vi "Length_14.vi"() -> ()   [LabVIEW 2020]
uses:
  Support/Controls/Cmd_Mouse Popup.ctl
  Support/Controls/Clst_Initialize Input.ctl
  Support/Controls/Cmd_Var Data IO.ctl
  Variables/Global_Cal Info.vi
  Support/Public/Polymorph/Rmv Empt Arr_1D Str.vi
  Support/Public/Polymorph/Data Class_2D Str.vi
  <vilib>/express/express arith-compare/Formula/XNode/ExpressFormulaBlockNode.xnode
panel:
  in  "dw조건":enum32{"큰 값", "가까운 값"}(radio)
  out "dw":string
  out "Force":string caption="측정력 참조"
  in  "측정력":string(combo)
  out "3 wire":string caption="3침 게이지"
  out "Resolution 2":string[][](table) caption="Spec"
  out "Resolution 1":string[][](table) caption="Spec"
  in  "형태":enum16{"GO/NOT GO", "GO", "NOT GO"}(ring) caption="나사형태"
  out "구분 2":string
  out "구분 1":string
  out "검색결과 2":string[](array[string])
  out "종류 2":string
  out "등급셋":string[][](array[string])
  out "검색결과 1":string[](array[string])
  out "종류셋":string[][][](array[string])
  out "규격셋":string[][](array[string])
  out "Spec 2":string[][](table) caption="Spec (명목 직경)"
  out "Condition 2":string[][](table) caption="2. 직경 측정결과"
  in  "Measured 2":string[][](table) caption="지시편차 (μm)"
  out "종류 1":string
  in  "등급":string(combo)
  in  "기호":string(combo)
  in  "피치or산 수":string(combo)
  in  "호칭치수":string(combo)
  in  "나사구분":string(combo)="M"
  in  "Spec 변경":bool
  in  "Random":bool
  out "Spec 1":string[][](table) caption="Spec (명목 직경)"
  out "제목":string
  out "에러 출력":errorcluster
  out "Condition 1":string[][](table) caption="2. 직경 측정결과"
  in  "Measured 1":string[][](table) caption="지시편차 (μm)"
  out "Load?":bool
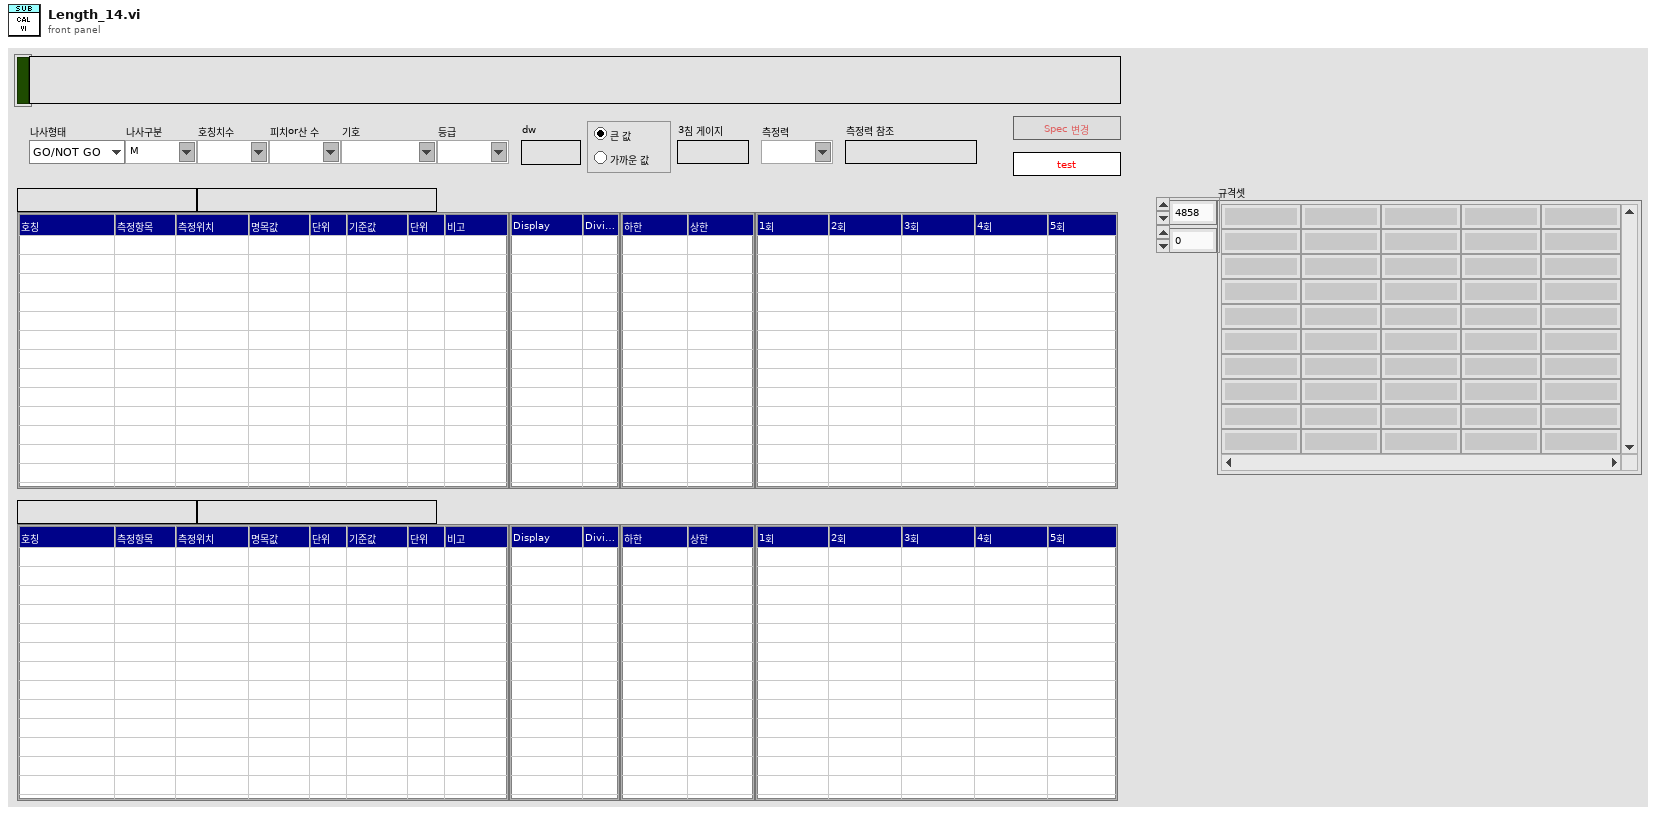
[diagram p1: front panel]
types:
  T1 = typedef "Cmd_Mouse Popup.ctl" = enum16{"활성화", "메뉴선택"}
  T2 = cluster{"Shift":bool, "Ctrl":bool, "Alt":bool, "Cmd":bool, "Opt":bool}
  T3 = typedef "Clst_Initialize Input.ctl" = cluster{"Initialize 1":cluster{"Condition":refnum<vi>[], "Spec":refnum<vi>[], "Measured":refnum<vi>[], "Resolution":refnum<vi>[], "Func_ext":string, "제목":refnum<vi>, "Measured_ADJ":refnum<vi>[]}, "Initialize 2":cluster{"문자열":refnum<vi>[], "콤보박스":refnum<vi>[], "링":refnum<vi>[], "열거형":refnum<vi>[], "테이블":refnum<vi>[], "여러열":refnum<vi>[], "디지털(DBL)":refnum<vi>[], "3D string":refnum<vi>[], "ctrl":refnum<vi>[], "boolean":refnum<vi>[]}}
  T4 = typedef "Cmd_Var Data IO.ctl" = enum16{"Condition", "Condition Default", "Condition_Temp", "Resolution", "Resolution Default", "Resolution Old", "Spec", "Spec Default", "Spec Old", "Spec Temp", "Result", "Result2", "Result3", "Result_Temp", "Result_ADJ", "Result_ADJ2", "STD1", "STD2", "STD3", "STD4", "STD5", "STD Temp", "CMC", "CMC Default"}
  T5 = typedef "LVComboBoxStrsAndValuesArrayTypeDef.ctl" = cluster{"String":string, "Value":string}[]
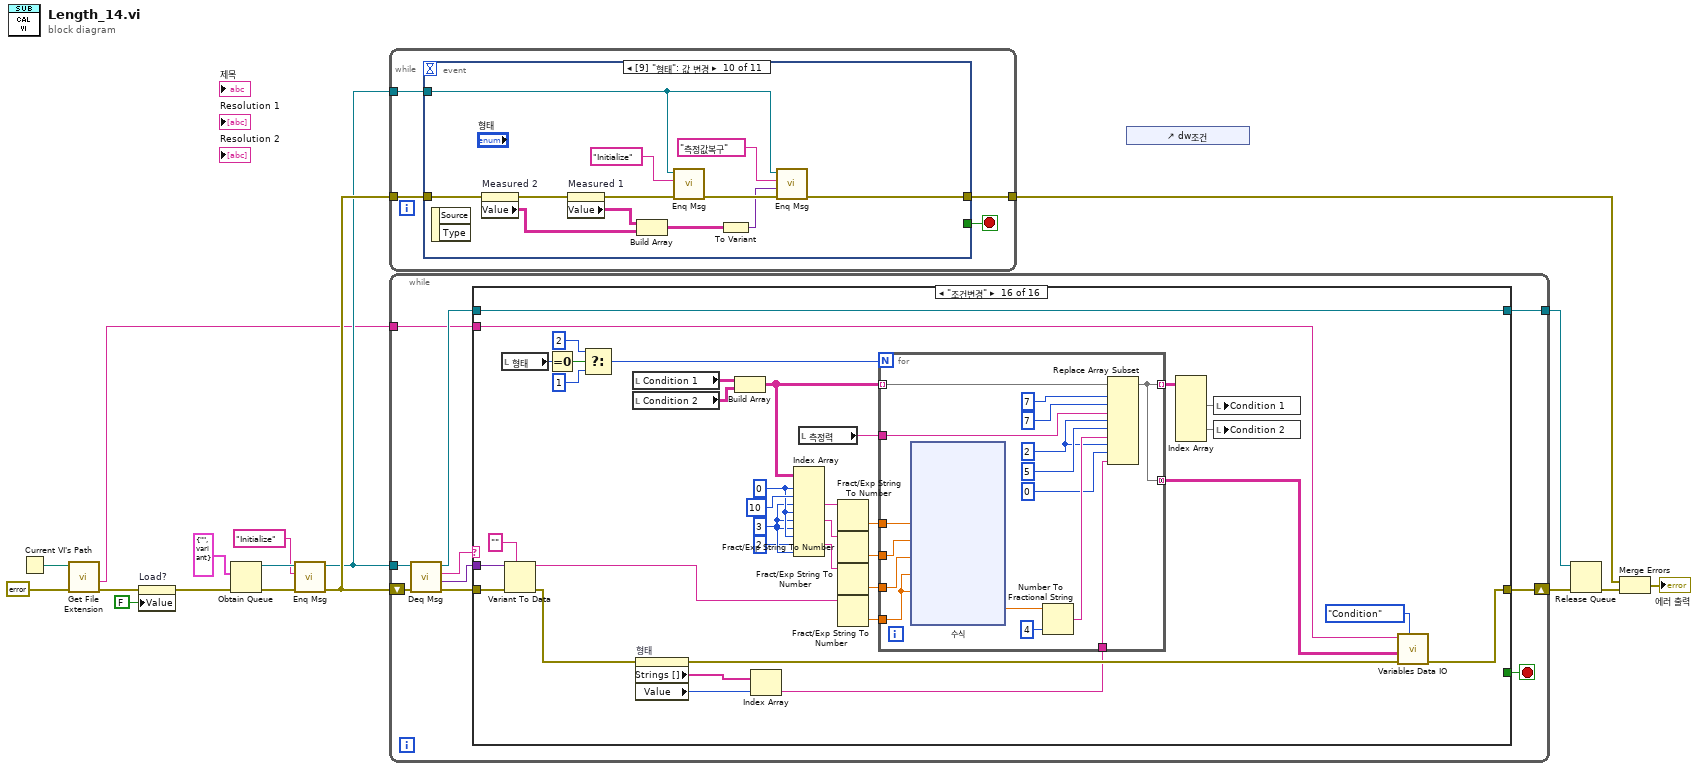
[diagram p0: block diagram]
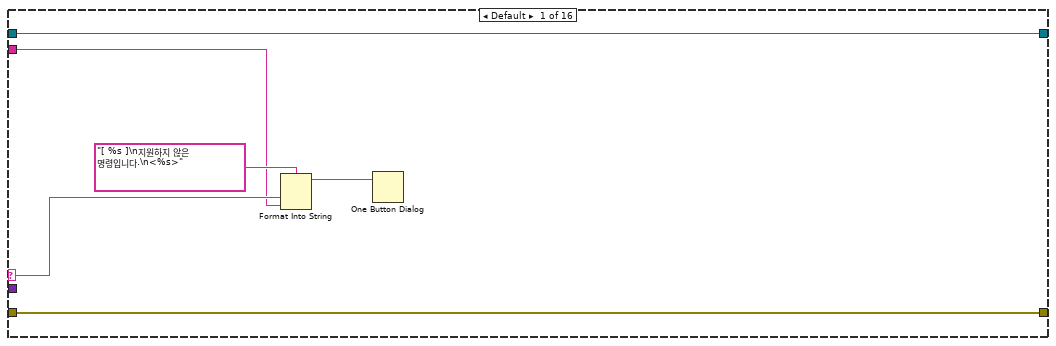
[diagram p2: hidden frame]
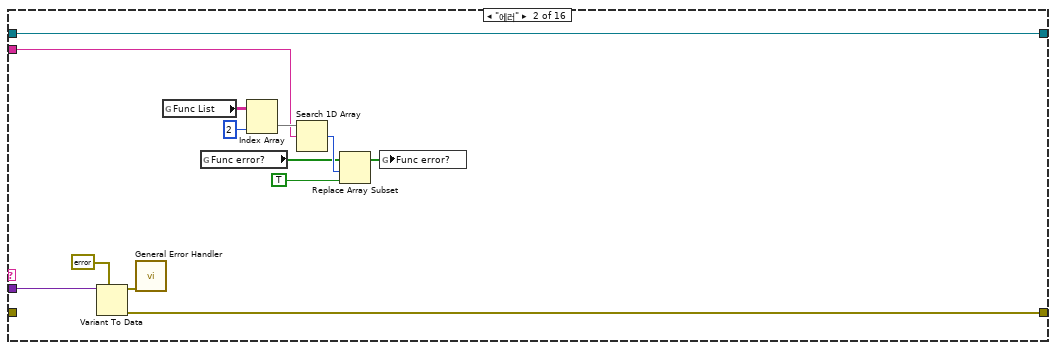
[diagram p3: hidden frame]
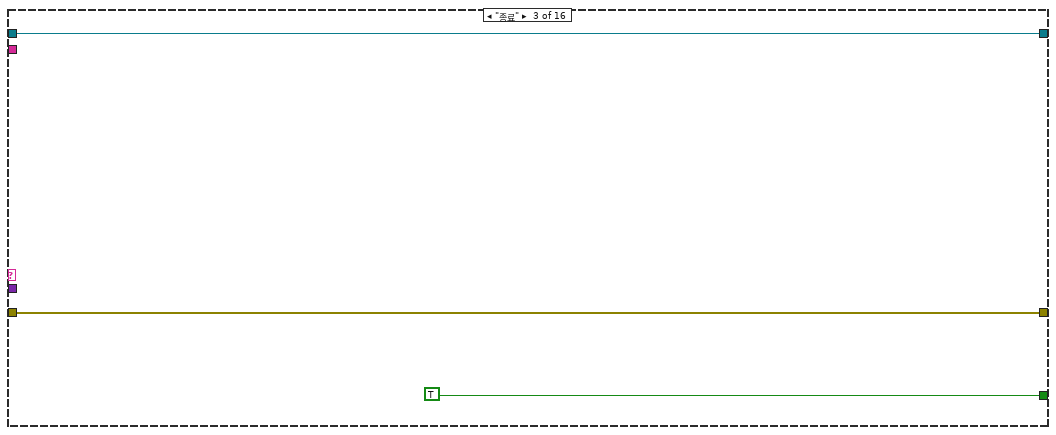
[diagram p4: hidden frame]
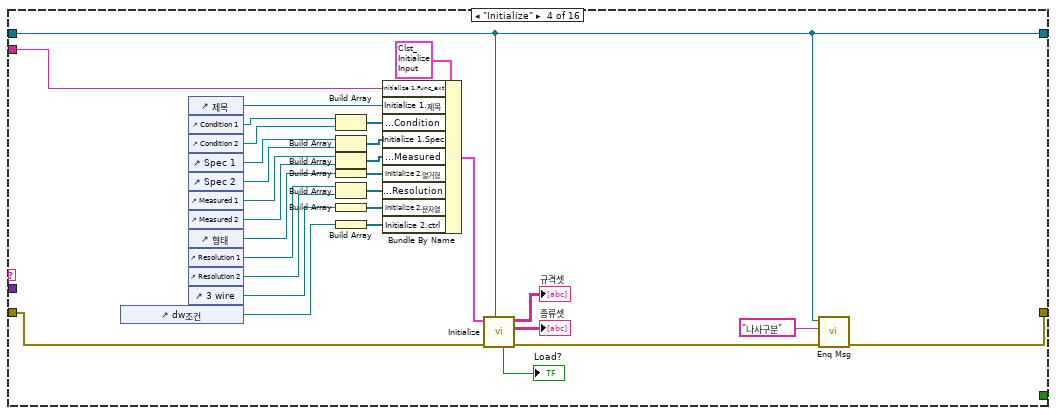
[diagram p5: hidden frame]
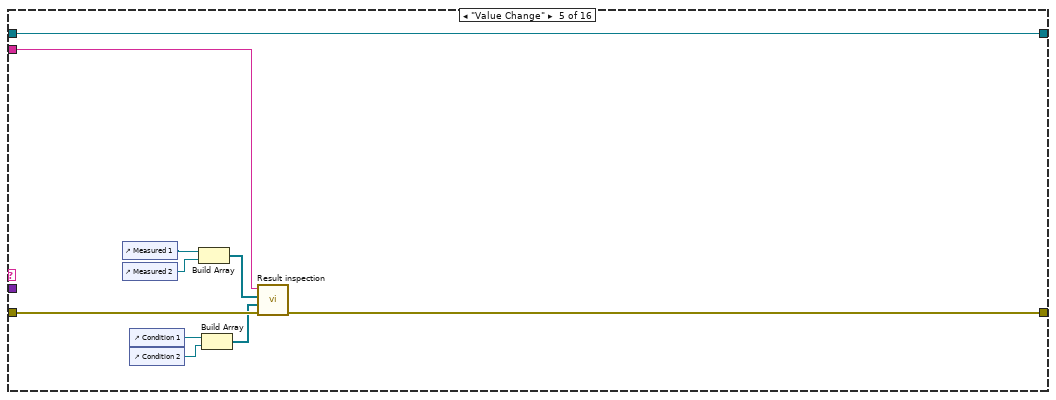
[diagram p6: hidden frame]
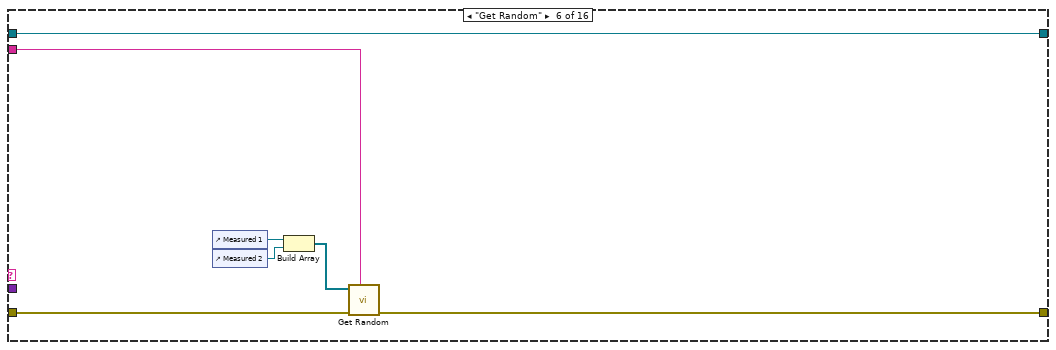
[diagram p7: hidden frame]
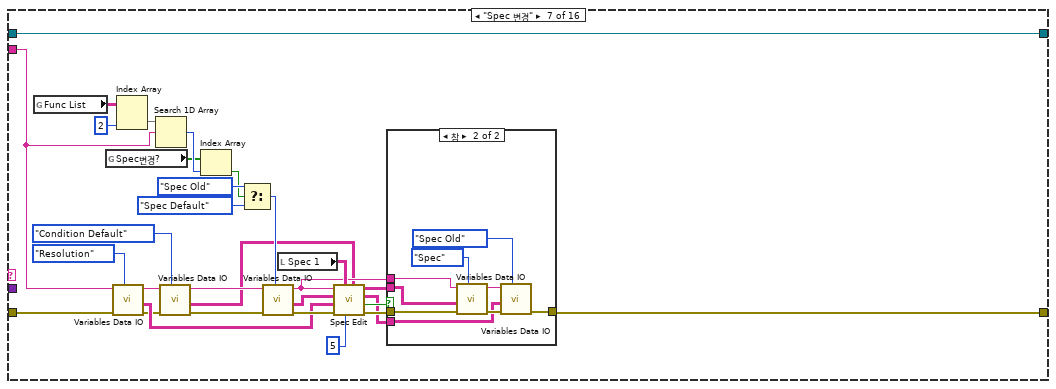
[diagram p8: hidden frame]
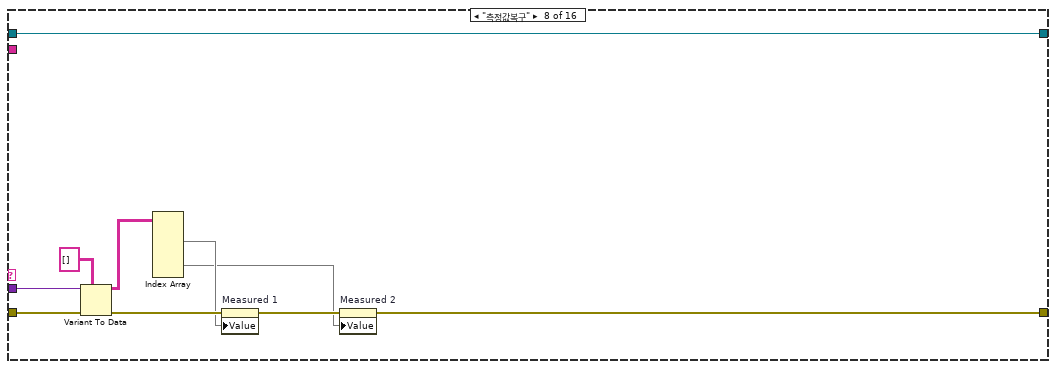
[diagram p10: hidden frame]
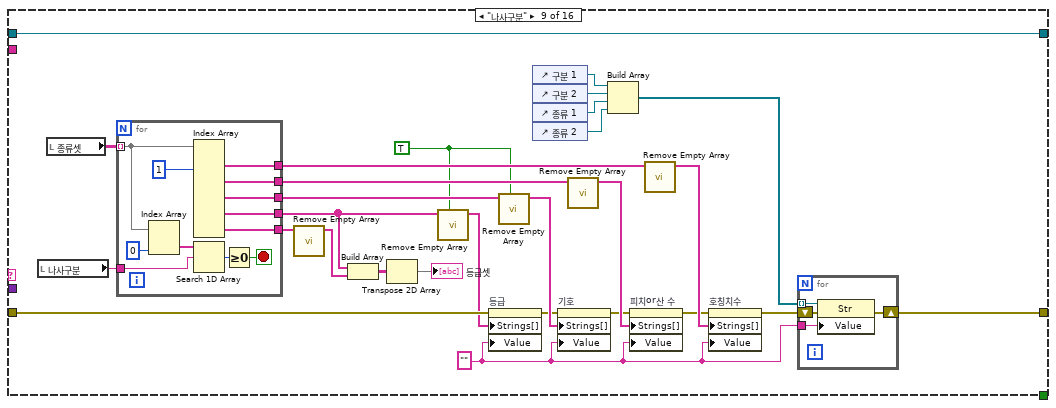
[diagram p11: hidden frame]
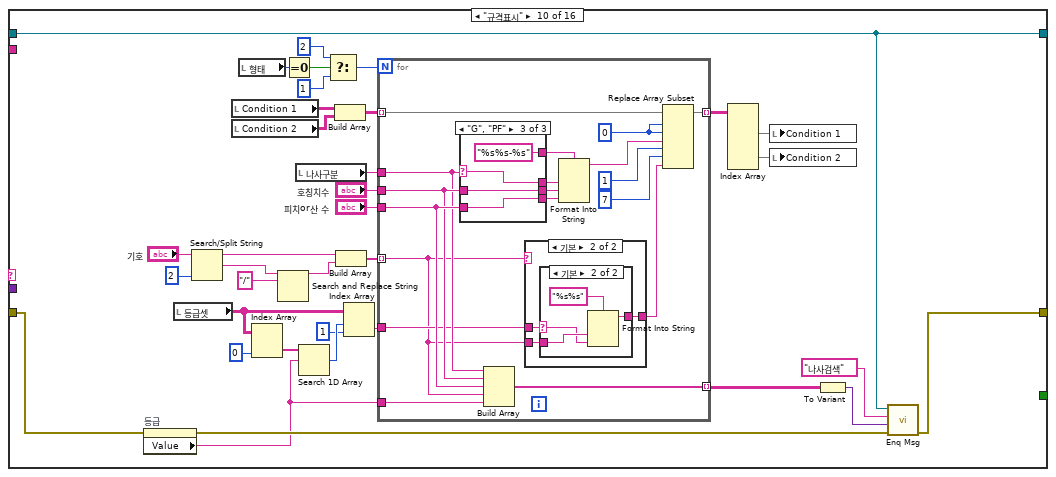
[diagram p12: hidden frame]
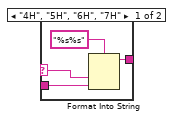
[diagram p14: hidden frame]
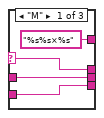
[diagram p15: hidden frame]
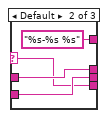
[diagram p16: hidden frame]
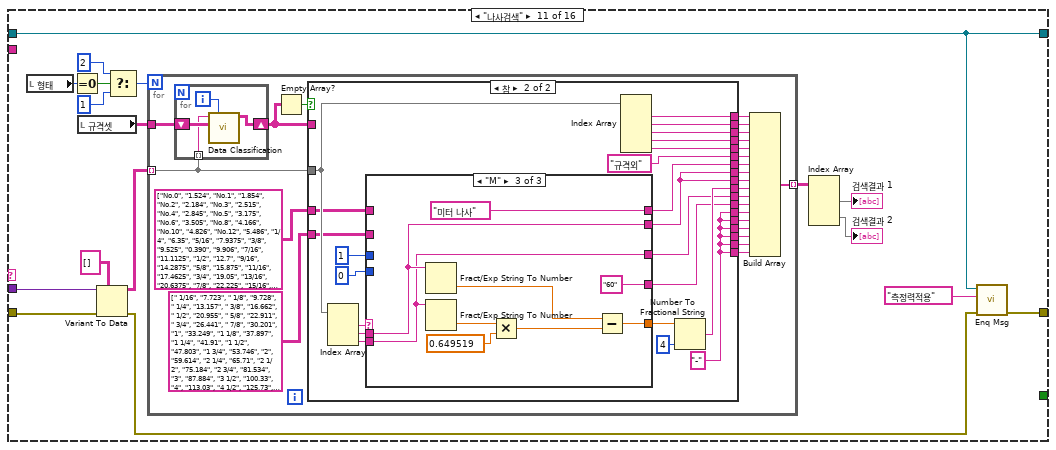
[diagram p17: hidden frame]
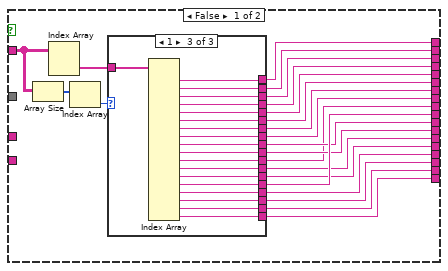
[diagram p18: hidden frame]
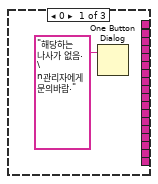
[diagram p19: hidden frame]
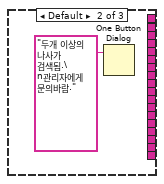
[diagram p20: hidden frame]
diagram:
  n1 = Current VI's Path() -> (path=w5:path)
  n2 = call <vilib>:"Get File Extension.vi"("error in (no error)"=errorcluster {"status"=FALSE, "code"=0, "source"=""} ("에러 상수"), "file"=w5) -> ("error out"=w3:errorcluster, "filename without extension"=w4:string)  [unwired: 5 in, 3 out]
  n3 = property on="Load?" class="Bool (엄격한)"(error in=w3, "Value"=FALSE ("Load?")) -> (error out=w2:errorcluster)  [unwired: 1 in, 1 out]
  n4 = Obtain Queue(element data type=cluster{"메세지":string, "값":variant} {"메세지"="", "값"=variant} ("Message Cluster"), error in (no error)=w2) -> (queue out=w14:refnum<queue>, error out=w16:errorcluster)  [unwired: 3 in, 1 out]
  n5 = call "Enq Msg.vi"("에러 입력(에러 없음)"=w16, "메세지"="Initialize", "큐 입력"=w14) -> ("에러 출력"=w15:errorcluster, "큐 출력"=w12:refnum<queue>)  [unwired: 7 in]
  n6 = while {
    tunnel: w15 -> [w19]
    tunnel: w12 -> [w20]
    tunnel: [w18] -> w9
    stop <- w21 stop-if-true
    n7 = event shown="[9] \"형태\": 값 변경" {
      selector: _ -> [_ _ _ _ _ _ _ _ _ _ _]
      dyn-events: _ -> [_ _ _ _ _ _ _ _ _ _ _]
      timeout: _ -> [_ _ _ _ _ _ _ _ _ _ _]
      tunnel: [w27 _ _ _ _ _ _ _ _ _ _] -> w21
      tunnel: w20 -> [w25 w31 _ w36 _ w54 w58 w61 w74 w94 w102]
      tunnel: w19 -> [w26 w29 w35 w43 w49 w55 w59 w64 w73 w92 w103]
      tunnel: [w23 w30 w34 w37 w48 w50 w57 w62 w76 w95 w101] -> w18
      event Panel Close? {
        w27 = TRUE ("버림?")
        n8 = event-data() -> ()  [unwired: 1 in, 1 out]
        n9 = call "Enq Msg.vi"("우선순위 메시지?"=TRUE, "에러 입력(에러 없음)"=w26, "메세지"="종료", "큐 입력"=w25) -> ("에러 출력"=w23:errorcluster)  [unwired: 6 in, 1 out]
        n10 = event-data("Discard?"=w27) -> ()  [unwired: 1 in, 1 out]
      }
      event "Measured 1", "Measured 2": Value Change {
        n11 = event-data() -> ()  [unwired: 1 in, 1 out]
        n12 = call "Enq Msg.vi"("에러 입력(에러 없음)"=w29, "메세지"="Value Change", "큐 입력"=w31) -> ("에러 출력"=w30:errorcluster)  [unwired: 7 in, 1 out]
      }
      event "Condition 1", "Spec 1", "Measured 1", "Condition 2", "Spec 2", "Measured 2": Shortcut Menu Activation? {
        n13 = event-data() -> ("MenuRef"=w33:refnum<k9>)  [unwired: 1 in]
        n14 = call "Mouse PopUp Control.vi"("type"=Cmd_Mouse_Popup."활성화", "error in"=w35, "메뉴 참조"=w33) -> ("error out"=w34:errorcluster)  [unwired: 8 in]
        n15 = event-data() -> ()  [unwired: 2 in, 1 out]
      }
      event "Condition 1", "Spec 1", "Measured 1", "Condition 2", "Spec 2", "Measured 2": Shortcut Menu Selection (User) {
        n16 = event-data() -> ("CtlRef"=w41:refnum<vi>, "ItemTag"=w40:string)  [unwired: 1 in]
        n17 = call "Mouse PopUp Control.vi"("type"=Cmd_Mouse_Popup."메뉴선택", "error in"=w43, "아이템 태그"=w40, "Tbl 참조 번호"=w41) -> ("error out"=w38:errorcluster)  [unwired: 7 in]
        n18 = call "Enq Msg.vi"("에러 입력(에러 없음)"=w38, "메세지"="Value Change", "큐 입력"=w36) -> ("에러 출력"=w37:errorcluster)  [unwired: 7 in, 1 out]
      }
      event "Measured 1", "Condition 1", "Measured 2", "Condition 2": Key Down; "Measured 1", "Condition 1", "Measured 2", "Condition 2": Key Repeat {
        n19 = event-data() -> ("PlatMods"=w44:T2, "ScanCode"=w47:i16, "Mods.Num Pad"=w46:bool, "CtlRef"=w45:refnum<vi>)  [unwired: 1 in]
        n20 = call "Cursor Control.vi"("플랫폼 조합키"=w44, "참조"=w45, "Num Pad"=w46, "ScanCode"=w47, "error in"=w49) -> ("error out"=w48:errorcluster)  [unwired: 5 in, 1 out]
      }
      event "Random": Value Change {
        n21 = event-data() -> ()  [unwired: 1 in, 1 out]
        n22 = call "Enq Msg.vi"("에러 입력(에러 없음)"=w55, "메세지"="Get Random", "큐 입력"=w54) -> ("에러 출력"=w53:errorcluster, "큐 출력"=w52:refnum<queue>)  [unwired: 7 in]
        n23 = call "Enq Msg.vi"("에러 입력(에러 없음)"=w53, "메세지"="Value Change", "큐 입력"=w52) -> ("에러 출력"=w50:errorcluster)  [unwired: 7 in, 1 out]
      }
      event "Spec 변경": Value Change {
        n24 = event-data() -> ()  [unwired: 1 in, 1 out]
        n25 = call "Enq Msg.vi"("에러 입력(에러 없음)"=w59, "메세지"="Spec 변경", "큐 입력"=w58) -> ("에러 출력"=w57:errorcluster)  [unwired: 7 in, 1 out]
      }
      event "나사구분": Value Change {
        n26 = event-data() -> ()  [unwired: 1 in, 2 out]
        n27 = call "Enq Msg.vi"("에러 입력(에러 없음)"=w64, "메세지"="나사구분", "큐 입력"=w61) -> ("에러 출력"=w62:errorcluster)  [unwired: 7 in, 1 out]
      }
      event "호칭치수", "피치or산 수", "등급", "기호", "dw조건": Value Change {
        n28 = event-data() -> ()  [unwired: 1 in, 2 out]
        n29 = call "Enq Msg.vi"("에러 입력(에러 없음)"=w73, "메세지"="규격표시", "큐 입력"=w74) -> ("에러 출력"=w76:errorcluster)  [unwired: 7 in, 1 out]
        n30 = local read "피치or산 수"() -> (w72:string)
        n31 = local read "나사구분"() -> (w71:string)
        n32 = Fract/Exp String To Number(string=w72) -> (number=w68:dbl)  [unwired: 3 in, 1 out]
        n33 = case shown="\"M\"" w71 {
          tunnel: [60.0 ("y") 55.0 ("y") 60.0 ("y")] -> w70
          tunnel: w68 -> [w77 w80 w84]
          tunnel: [w77 w79 w83] -> w69
          frame "M" {
          }
          frame "G", "PF" {
            n34 = Divide(x=25.4 ("y"), y=w80) -> (x/y=w79:dbl)
          }
          frame Default {
            n35 = Divide(x=25.4 ("y"), y=w84) -> (x/y=w83:dbl)
          }
        }
        n36 = call "Thread_dw.vi"("α"=w70, "P"=w69) -> ("결과"=w67:dbl)  [unwired: 1 in, 1 out]
        n37 = Number To Fractional String(number=w67, precision (6)=i16 4 ("정밀도(6)")) -> (F-format string=→"dw":string)  [unwired: 2 in]
      }
      event "형태": Value Change {
        n38 = event-data() -> ()  [unwired: 1 in, 2 out]
        n39 = property on="Measured 2" class="Tbl (엄격한)"(error in=w92) -> (error out=w91:errorcluster, "Value"=w89:string[][])  [unwired: 1 in, 1 out]
        n40 = property on="Measured 1" class="Tbl (엄격한)"(error in=w91) -> (error out=w90:errorcluster, "Value"=w88:string[][])  [unwired: 1 in, 1 out]
        n41 = Build Array(w88, w89) -> (w87:string[][][])
        n42 = call "Enq Msg.vi"("에러 입력(에러 없음)"=w90, "메세지"="Initialize", "큐 입력"=w94) -> ("에러 출력"=w96:errorcluster)  [unwired: 7 in, 1 out]
        n43 = To Variant(anything=w87) -> (Variant=w93:variant)
        n44 = call "Enq Msg.vi"("에러 입력(에러 없음)"=w96, "값"=w93, "메세지"="측정값복구", "큐 입력"=w94) -> ("에러 출력"=w95:errorcluster)  [unwired: 6 in, 1 out]
      }
      event "측정력": Value Change {
        n45 = event-data() -> ()  [unwired: 1 in, 2 out]
        n46 = To Variant(anything="측정력") -> (Variant=w99:variant)
        n47 = call "Enq Msg.vi"("에러 입력(에러 없음)"=w103, "값"=w99, "메세지"="조건변경", "큐 입력"=w102) -> ("에러 출력"=w101:errorcluster)  [unwired: 6 in, 1 out]
      }
    }
  }
  n48 = while {
    shift-right: [w114] -> w11
    shift-left: w15 -> [w113]
    tunnel: w12 -> [w111]
    tunnel: [w106] -> w10
    tunnel: w4 -> [w105]
    stop <- w107 stop-if-true
    n49 = call "Deq Msg.vi"("에러 입력(에러 없음)"=w113, "큐 입력"=w111) -> ("에러 출력"=w112:errorcluster, "값"=w108:variant, "메세지"=w110:string, "큐 출력"=w109:refnum<queue>)  [unwired: 6 in]
    n50 = case shown="\"조건변경\"" w110 {
      selector: w110 -> [w116 _ _ _ _ _ _ _ _ _ _ _ _ _ _ _]
      tunnel: w112 -> [w120 _ w136 w166 w171 w179 w206 w230 w250 w306 w370 w549 w577 w683 w840 w898]
      tunnel: [w120 w130 w136 w148 w175 w180 w209 w225 w245 w311 w365 w544 w603 w675 w811 w892] -> w114
      tunnel: w109 -> [w119 w129 w134 w147 w176 w183 w213 w233 w261 w302 w364 w543 w602 w674 w810 w907]
      tunnel: w108 -> [_ w131 _ _ _ _ _ w231 _ _ w369 _ w576 _ _ w897]
      tunnel: [_ _ TRUE ("버림?") _ _ _ _ _ _ _ _ _ _ _ _ _] -> w107
      tunnel: [w119 w129 w134 w147 w176 w183 w213 w233 w261 w302 w364 w543 w602 w674 w810 w907] -> w106
      tunnel: w105 -> [w115 w121 _ w156 w174 w178 w191 _ _ _ _ _ _ w682 w835 w891]
      frame Default {
        n51 = Format Into String(format string="[ %s ]\n지원하지 않은 명령입니다.\n<%s>" ("메시지"), w116, w115) -> (resulting string=w117:string)  [unwired: 2 in, 1 out]
        n52 = One Button Dialog(message=w117) -> ()  [unwired: 1 in, 1 out]
      }
      frame "에러" {
        n53 = Variant To Data(type=errorcluster {"status"=FALSE, "code"=0, "source"=""} ("에러 출력"), Variant=w131) -> (data=w133:errorcluster, error out=w130:errorcluster)  [unwired: 1 in]
        n54 = call <vilib>:"General Error Handler.vi"("error in (no error)"=w133) -> ()  [unwired: 10 in, 5 out]
        n55 = global read "Global_Cal Info.vi" "Func List"() -> (w123:string[][])
        n56 = global read "Global_Cal Info.vi" "Func error?"() -> (w126:bool[])
        n57 = Index Array(array=w123, index (col)=2 ("비활성화된 인덱스 (열)")) -> (element=w124:string[])  [unwired: 1 in]
        n58 = Search 1D Array(1D array=w124, element=w121) -> (index of element=w127:i32)  [unwired: 1 in]
        n59 = Replace Array Subset(array=w126, new element=TRUE ("새 원소/부분배열"), index=w127) -> (w128:bool[])
        n60 = global write "Global_Cal Info.vi" "Func error?"(w128) -> ()
      }
      frame "종료" {
      }
      frame "Initialize" {
        n61 = control-ref of="dw조건"() -> (w138:refnum<vi>)
        n62 = control-ref of="제목"() -> (w159:refnum<vi>)
        n63 = control-ref of="Condition 1"() -> (w163:refnum<vi>)
        n64 = control-ref of="Condition 2"() -> (w154:refnum<vi>)
        n65 = control-ref of="Spec 1"() -> (w158:refnum<vi>)
        n66 = control-ref of="Spec 2"() -> (w153:refnum<vi>)
        n67 = control-ref of="Measured 1"() -> (w160:refnum<vi>)
        n68 = control-ref of="Measured 2"() -> (w152:refnum<vi>)
        n69 = control-ref of="형태"() -> (w146:refnum<vi>)
        n70 = control-ref of="Resolution 1"() -> (w144:refnum<vi>)
        n71 = control-ref of="Resolution 2"() -> (w143:refnum<vi>)
        n72 = control-ref of="3 wire"() -> (w140:refnum<vi>)
        n73 = Build Array(w163, w154) -> (w162:refnum<vi>[])
        n74 = Build Array(w158, w153) -> (w157:refnum<vi>[])
        n75 = Build Array(w160, w152) -> (w161:refnum<vi>[])
        n76 = Build Array(w146) -> (w145:refnum<vi>[])
        n77 = Build Array(w144, w143) -> (w142:refnum<vi>[])
        n78 = Build Array(w140) -> (w139:refnum<vi>[])
        n79 = Build Array(w138) -> (w137:refnum<vi>[])
        n80 = Bundle By Name(cluster=T3 {"Initialize 1"={"Condition"=[], "Spec"=[], "Measured"=[], "Resolution"=[], "Func_ext"="", "제목"=refnum, "Measured_ADJ"=[]}, "Initialize 2"={"문자열"=[], "콤보박스"=[], "링"=[], "열거형"=[], "테이블"=[], "여러열"=[], "디지털(DBL)"=[], "3D string"=[], "ctrl"=[], "boolean"=[]}} ("입력 클러스터"), "Initialize 1.Func_ext"=w156, "Initialize 1.제목"=w159, "Initialize 1.Condition"=w162, "Initialize 1.Spec"=w157, "Initialize 1.Measured"=w161, "Initialize 2.열거형"=w145, "Initialize 1.Resolution"=w142, "Initialize 2.문자열"=w139, "Initialize 2.ctrl"=w137) -> (w164:T3)
        n81 = call "Initialize.vi"("큐 입력"=w147, "error in"=w166, "입력 클러스터"=w164) -> ("error out"=w149:errorcluster, "data 2 (3d)"=→"종류셋":string[][][], "data 1 (2d)"=→"규격셋":string[][], "Load?"=→"Load?":bool)  [unwired: 5 in]
        n82 = call "Enq Msg.vi"("에러 입력(에러 없음)"=w149, "메세지"="나사구분", "큐 입력"=w147) -> ("에러 출력"=w148:errorcluster)  [unwired: 7 in, 1 out]
      }
      frame "Value Change" {
        n83 = control-ref of="Measured 1"() -> (w173:refnum<vi>)
        n84 = control-ref of="Measured 2"() -> (w170:refnum<vi>)
        n85 = control-ref of="Condition 1"() -> (w169:refnum<vi>)
        n86 = control-ref of="Condition 2"() -> (w168:refnum<vi>)
        n87 = Build Array(w173, w170) -> (w172:refnum<vi>[])
        n88 = Build Array(w169, w168) -> (w167:refnum<vi>[])
        n89 = call "Result inspection.vi"("error in"=w171, "Ref. Data (excluded)"=w167, "Ref. Data (Inspection)"=w172, "Func ext"=w174) -> ("error out"=w175:errorcluster)  [unwired: 4 in, 3 out]
      }
      frame "Get Random" {
        n90 = control-ref of="Measured 1"() -> (w182:refnum<vi>)
        n91 = control-ref of="Measured 2"() -> (w177:refnum<vi>)
        n92 = Build Array(w182, w177) -> (w181:refnum<vi>[])
        n93 = call "Get Random.vi"("Func_Ext"=w178, "에러 입력"=w179, "Meas"=w181) -> ("에러 출력"=w180:errorcluster)  [unwired: 7 in, 1 out]
      }
      frame "Spec 변경" {
        n94 = global read "Global_Cal Info.vi" "Func List"() -> (w196:string[][])
        n95 = global read "Global_Cal Info.vi" "Spec변경?"() -> (w192:bool[])
        n96 = call "Variables Data IO.vi"("Select"=Cmd_Var_Data_IO."Resolution", "error in"=w206, "Func_ext"=w191) -> ("error out"=w189:errorcluster, "Data Out"=w200:string[][], "Func_ext Out"=w187:string)  [unwired: 6 in]
        n97 = Index Array(array=w196, index (col)=2 ("비활성화된 인덱스 (열)")) -> (element=w194:string[])  [unwired: 1 in]
        n98 = Search 1D Array(1D array=w194, element=w191) -> (index of element=w193:i32)  [unwired: 1 in]
        n99 = call "Variables Data IO.vi"("Select"=Cmd_Var_Data_IO."Condition Default", "error in"=w189, "Func_ext"=w187) -> ("error out"=w188:errorcluster, "Data Out"=w184:string[][], "Func_ext Out"=w186:string)  [unwired: 6 in]
        n100 = Index Array(array=w192, index=w193) -> (element=w197:bool)
        n101 = Select(t=Cmd_Var_Data_IO."Spec Old" ("Select"), s=w197, f=Cmd_Var_Data_IO."Spec Default" ("Select")) -> (s? t:f=w190:T4)
        n102 = call "Variables Data IO.vi"("Select"=w190, "error in"=w188, "Func_ext"=w186) -> ("error out"=w208:errorcluster, "Data Out"=w201:string[][], "Func_ext Out"=w202:string)  [unwired: 6 in]
        n103 = local read "Spec 1"() -> (w203:string[][])
        n104 = call "Spec Edit.vi"("Condition"=w184, "열번호(기준값)"=5, "Spec Value"=w203, "에러 입력(에러 없음)"=w208, "Resolution"=w200, "Spec Default"=w201, "Func_ext"=w202) -> ("에러 출력"=w210:errorcluster, "변경?"=w211:bool, "Spec Default out"=w205:string[][], "Spec 출력"=w212:string[][])  [unwired: 1 in]
        n105 = case shown="참" w211 {
          tunnel: w212 -> [_ w215]
          tunnel: w210 -> [w214 w223]
          tunnel: [w214 w219] -> w209
          tunnel: w202 -> [_ w221]
          tunnel: w205 -> [_ w217]
          frame False {
          }
          frame True {
            n106 = call "Variables Data IO.vi"("Select"=Cmd_Var_Data_IO."Spec", "error in"=w223, "Data In"=w215, "Func_ext"=w221) -> ("error out"=w220:errorcluster, "Func_ext Out"=w218:string)  [unwired: 5 in, 1 out]
            n107 = call "Variables Data IO.vi"("Select"=Cmd_Var_Data_IO."Spec Old", "error in"=w220, "Data In"=w217, "Func_ext"=w218) -> ("error out"=w219:errorcluster)  [unwired: 5 in, 2 out]
          }
        }
      }
      frame "측정값복구" {
        n108 = Variant To Data(error in=w230, type=string[][][] [], Variant=w231) -> (data=w228:string[][][], error out=w229:errorcluster)
        n109 = Index Array(array=w228) -> (element #1=w227:string[][], element #2=w224:string[][])  [unwired: 6 in]
        n110 = property on="Measured 1" class="Tbl (엄격한)"(error in=w229, "Value"=w227) -> (error out=w226:errorcluster)  [unwired: 1 in, 1 out]
        n111 = property on="Measured 2" class="Tbl (엄격한)"(error in=w226, "Value"=w224) -> (error out=w225:errorcluster)  [unwired: 1 in, 1 out]
      }
      frame "나사구분" {
        w234 = TRUE ("0번 공란삽입(F)")
        w244 = ""
        n112 = local read "나사구분"() -> (w260:string)
        n113 = local read "종류셋"() -> (w251:string[][][])
        n114 = for {
          tunnel: w251 -> [w272] mode=indexing
          tunnel: w260 -> [w275]
          tunnel: [w271] -> w254
          tunnel: [w270] -> w253
          tunnel: [w269] -> w252
          tunnel: [w268] -> w237
          tunnel: [w266] -> w247
          stop <- w273 stop-if-true
          n115 = Index Array(array=w272, index (col)=0 ("비활성화된 인덱스 (열)")) -> (element=w276:string[])  [unwired: 1 in]
          n116 = Index Array(array=w272, index (col) #1=1 ("비활성화된 인덱스 (열)")) -> (element #1=w271:string[], element #2=w270:string[], element #3=w269:string[], element #4=w268:string[], element #5=w266:string[])  [unwired: 9 in]
          n117 = Search 1D Array(1D array=w276, element=w275) -> (index of element=w274:i32)  [unwired: 1 in]
          n118 = Greater Or Equal To 0?(x=w274) -> (x >= 0?=w273:bool)
        }
        n119 = call-poly "Remove Empty Array.vi"("Data in"=w247) -> ("Data out"=w238:string[])  [unwired: 9 in, 1 out]
        n120 = Build Array(w237, w238) -> (w236:string[][])
        n121 = Transpose 2D Array(2D array=w236) -> (transposed array=→"등급셋":string[][])
        n122 = call-poly "Remove Empty Array.vi"("0번 공란삽입(F)"=w234, "Data in"=w237) -> ("Data out"=w248:string[])  [unwired: 8 in, 1 out]
        n123 = property on="등급" class="CmbBox"(error in=w250, "Strings[]"=w248, "Value"=w244) -> (error out=w249:errorcluster)  [unwired: 1 in, 1 out]
        n124 = call-poly "Remove Empty Array.vi"("0번 공란삽입(F)"=w234, "Data in"=w252) -> ("Data out"=w259:string[])  [unwired: 8 in, 1 out]
        n125 = control-ref of="구분 1"() -> (w243:refnum<vi>)
        n126 = control-ref of="구분 2"() -> (w242:refnum<vi>)
        n127 = control-ref of="종류 1"() -> (w241:refnum<vi>)
        n128 = control-ref of="종류 2"() -> (w240:refnum<vi>)
        n129 = property on="기호" class="CmbBox"(error in=w249, "Strings[]"=w259, "Value"=w244) -> (error out=w257:errorcluster)  [unwired: 1 in, 1 out]
        n130 = call-poly "Remove Empty Array.vi"("Data in"=w253) -> ("Data out"=w258:string[])  [unwired: 9 in, 1 out]
        n131 = Build Array(w243, w242, w241, w240) -> (w239:refnum<vi>[])
        n132 = property on="피치or산 수" class="CmbBox"(error in=w257, "Strings[]"=w258, "Value"=w244) -> (error out=w255:errorcluster)  [unwired: 1 in, 1 out]
        n133 = call-poly "Remove Empty Array.vi"("Data in"=w254) -> ("Data out"=w256:string[])  [unwired: 9 in, 1 out]
        n134 = property on="호칭치수" class="CmbBox"(error in=w255, "Strings[]"=w256, "Value"=w244) -> (error out=w246:errorcluster)  [unwired: 1 in, 1 out]
        n135 = for {
          shift-right: [w264] -> w245
          shift-left: w246 -> [w265]
          tunnel: w244 -> [w263]
          tunnel: w239 -> [w262] mode=indexing
          n136 = property class="Str"(reference=w262, error in=w265, "Value"=w263) -> (error out=w264:errorcluster)  [unwired: 1 out]
        }
      }
      frame "규격표시" {
        n137 = property on="등급" class="CmbBox"(error in=w306) -> (error out=w305:errorcluster, "Value"=w298:string)  [unwired: 1 in, 1 out]
        n138 = local read "등급셋"() -> (w289:string[][])
        n139 = Search/Split String(string="기호", offset (0)=2 ("오프셋(0)")) -> (substring before match=w297:string, match + rest of string=w280:string)  [unwired: 1 in, 1 out]
        n140 = local read "Condition 1"() -> (w295:string[][])
        n141 = local read "Condition 2"() -> (w294:string[][])
        n142 = local read "형태"() -> (w285:enum16{"GO/NOT GO", "GO", "NOT GO"})
        n143 = Index Array(array=w289, index (col)=0 ("비활성화된 인덱스 (열)")) -> (element=w287:string[])  [unwired: 1 in]
        n144 = Search and Replace String(input string=w280, search string="/" ("검색 문자열")) -> (result string=w279:string)  [unwired: 6 in, 3 out]
        n145 = Equal To 0?(x=w285) -> (x = 0?=w284:bool)
        n146 = local read "나사구분"() -> (w307:string)
        n147 = Search 1D Array(1D array=w287, element=w298) -> (index of element=w310:i32)  [unwired: 1 in]
        n148 = Select(t=2, s=w284, f=1) -> (s? t:f=w281:i32)
        n149 = Build Array(w295, w294) -> (w293:string[][][])
        n150 = Build Array(w297, w279) -> (w296:string[])
        n151 = Index Array(array=w289, index (row)=w310, index (col)=1 ("비활성화된 인덱스 (열)")) -> (element=w301:string)
        n152 = for {
          N: w281 -> [_]
          tunnel: "피치or산 수" -> [w330]
          tunnel: "호칭치수" -> [w329]
          tunnel: [w323] -> w303 mode=indexing
          tunnel: w301 -> [w322]
          tunnel: w298 -> [w321]
          tunnel: w296 -> [w313] mode=indexing
          tunnel: w307 -> [w324]
          tunnel: w293 -> [w320] mode=indexing
          tunnel: [w317] -> w292 mode=indexing
          w319 = 0 ("인덱스 (행)")
          n153 = case shown="\"G\", \"PF\"" w324 {
            selector: w324 -> [w345 w346 w352]
            tunnel: w329 -> [w344 w348 w351]
            tunnel: w330 -> [w343 w347 w350]
            tunnel: ["%s%s×%s" ("포맷 문자열") "%s-%s %s" ("포맷 문자열") "%s%s-%s" ("포맷 문자열")] -> w325
            tunnel: [w345 w348 w352] -> w326
            tunnel: [w344 w347 w351] -> w327
            tunnel: [w343 w346 w350] -> w328
            frame "M" {
            }
            frame Default {
            }
            frame "G", "PF" {
            }
          }
          n154 = Build Array(w324, w329, w330, w313, w321) -> (w323:string[])
          n155 = case shown="기본" w313 {
            tunnel: w322 -> [_ w333]
            tunnel: w313 -> [_ w332]
            tunnel: [_ w331] -> w314
            frame "" {
            }
            frame Default {
              n156 = case shown="기본" w333 {
                selector: w333 -> [w335 w339]
                tunnel: [w337 w341] -> w331
                tunnel: w332 -> [w336 w340]
                frame "4H", "5H", "6H", "7H" {
                  n157 = Format Into String(format string="%s%s", w335, w336) -> (resulting string=w337:string)  [unwired: 2 in, 1 out]
                }
                frame Default {
                  n158 = Format Into String(format string="%s%s", w340, w339) -> (resulting string=w341:string)  [unwired: 2 in, 1 out]
                }
              }
            }
          }
          n159 = Format Into String(format string=w325, w326, w327, w328) -> (resulting string=w318:string)  [unwired: 2 in, 1 out]
          n160 = Replace Array Subset(array=w320, new element #1=w318, index (row) #1=w319, index (col) #1=w319, new element #2=w314, index (row) #2=1 ("인덱스 (행)"), index (col) #2=7 ("인덱스 (행)")) -> (w317:string[][])
        }
        n161 = Index Array(array=w292) -> (element #1=w291:string[][], element #2=w290:string[][])  [unwired: 6 in]
        n162 = local write "Condition 1"(w291) -> ()
        n163 = local write "Condition 2"(w290) -> ()
        n164 = To Variant(anything=w303) -> (Variant=w304:variant)
        n165 = call "Enq Msg.vi"("에러 입력(에러 없음)"=w305, "값"=w304, "메세지"="나사검색", "큐 입력"=w302) -> ("에러 출력"=w311:errorcluster)  [unwired: 6 in, 1 out]
      }
      frame "나사검색" {
        n166 = local read "형태"() -> (w358:enum16{"GO/NOT GO", "GO", "NOT GO"})
        n167 = Equal To 0?(x=w358) -> (x = 0?=w357:bool)
        n168 = local read "규격셋"() -> (w367:string[][])
        n169 = Variant To Data(error in=w370, type=string[][] [], Variant=w369) -> (data=w362:string[][], error out=w366:errorcluster)
        n170 = Select(t=2, s=w357, f=1) -> (s? t:f=w354:i32)
        n171 = for {
          N: w354 -> [_]
          tunnel: w367 -> [w395]
          tunnel: [w383] -> w361 mode=indexing
          tunnel: w362 -> [w390] mode=indexing
          n172 = for {
            tunnel: w390 -> [w518] mode=indexing
            shift-right: [w519] -> w393
            shift-left: w395 -> [w521]
            i -> [w520]
            n173 = call-poly "Data Classification.vi"("인덱스"=w520, "DATA 입력"=w521, "검색 문자열"=w518) -> ("DATA 출력"=w519:string[][])  [unwired: 4 in, 4 out]
          }
          n174 = Empty Array?(array=w393) -> (empty?=w394:bool)
          n175 = case shown="참" w394 {
            tunnel: w393 -> [w414 _]
            tunnel: w390 -> [_ w455]
            tunnel: string[][] [["No.0", "1.524"], ["No.1", "1.854"], ["No.2", "2.184"], ["No.3", "2.515"], ["No.4", "2.845"], ["No.5", "3.175"], ["No.6", "3.505"], ["No.8", "4.166"], ["No.10", "4.826"], ["No.12", "5.486"], ["1/4", "6.35"], ["5/16", "7.9375"], ["3/8", "9.525"], ["0.390", "9.906"], ["7/16", "11.1125"], ["1/2", "12.7"], ["9/16", "14.2875"], ["5/8", "15.875"], ["11/16", "17.4625"], ["3/4", "19.05"], ["13/16", "20.6375"], ["7/8", "22.225"], ["15/16", "23.8125"], ["1", "25.4"], ["1 1/16", "26.9875"], ["1 1/8", "28.575"], ["1 3/16", "30.1625"], ["1 1/4", "31.75"], ["1 5/16", "33.3375"], ["1 3/8", "34.925"], ["1 7/16", "36.5125"], ["1 1/2", "38.1"], ["1 9/16", "39.6875"], ["1 5/8", "41.275"], ["1 11/16", "42.8625"], ["1 3/4", "44.45"], ["1 13/16", "46.0375"], ["1 7/8", "47.625"], ["1 15/16", "49.2125"], ["2", "50.8"], ["2 1/16", "52.3875"], ["2 1/8", "53.975"], ["2 3/16", "55.5625"], ["2 1/4", "57.15"], ["2 5/16", "58.7375"], ["2 3/8", "60.325"], ["2 7/16", "61.9125"], ["2 1/2", "63.5"], ["2 5/8", "66.675"], ["2 3/4", "69.85"], ["2 7/8", "73.025"], ["3", "76.2"], ["3 1/8", "79.375"], ["3 1/4", "82.55"], ["3 3/8", "85.725"], ["3 1/2", "88.9"], ["3 5/8", "92.075"], ["3 3/4", "95.25"], ["3 7/8", "98.425"], ["4", "101.6"], ["4 1/8", "104.775"], ["4 1/4", "107.95"], ["4 3/8", "111.125"], ["4 1/2", "114.3"], ["4 5/8", "117.475"], ["4 3/4", "120.65"], ["4 7/8", "123.825"], ["5", "127"], ["5 1/8", "130.175"], ["5 1/4", "133.35"], ["5 3/8", "136.525"], ["5 1/2", "139.7"], ["5 5/8", "142.875"], ["5 3/4", "146.05"], ["5 7/8", "149.225"], ["6", "152.4"]] ("테이블 컨트롤") -> [_ w450]
            tunnel: string[][] [[" 1/16", "7.723"], [" 1/8", "9.728"], [" 1/4", "13.157"], [" 3/8", "16.662"], [" 1/2", "20.955"], [" 5/8", "22.911"], [" 3/4", "26.441"], [" 7/8", "30.201"], ["1", "33.249"], ["1 1/8", "37.897"], ["1 1/4", "41.91"], ["1 1/2", "47.803"], ["1 3/4", "53.746"], ["2", "59.614"], ["2 1/4", "65.71"], ["2 1/2", "75.184"], ["2 3/4", "81.534"], ["3", "87.884"], ["3 1/2", "100.33"], ["4", "113.03"], ["4 1/2", "125.73"], ["5", "138.43"], ["5 1/2", "151.13"], ["6", "163.83"], ["7", "189.23"], ["8", "214.63"], ["9", "240.03"], ["10", "265.43"], ["12", "316.23"]] ("테이블 컨트롤") -> [_ w449]
            tunnel: [w412 w442] -> w389
            tunnel: [w411 "규격외" ("문자열")] -> w388
            tunnel: [w410 w441] -> w387
            tunnel: [w409 w440] -> w386
            tunnel: [w397 w440] -> w385
            tunnel: [w415 w454] -> w384
            tunnel: [w408 w453] -> w382
            tunnel: [w407 w452] -> w381
            tunnel: [w406 w451] -> w380
            tunnel: [w405 w451] -> w379
            tunnel: [w404 w451] -> w378
            tunnel: [w403 w451] -> w377
            tunnel: [w402 w451] -> w376
            tunnel: [w401 w451] -> w375
            tunnel: [w400 w443] -> w374
            tunnel: [w399 w445] -> w373
            tunnel: [w398 w444] -> w372
            tunnel: [w396 w446] -> w371
            frame False {
              n176 = Array Size(array=w414) -> (size(s)=w417:i32[])
              n177 = Index Array(array=w414) -> (element=w413:string[])  [unwired: 2 in]
              n178 = Index Array(array=w417) -> (element=w416:i32)  [unwired: 1 in]
              n179 = case shown="1" w416 {
                tunnel: [_ _ w421] -> w415
                tunnel: w413 -> [_ _ w438]
                tunnel: [_ _ w437] -> w412
                tunnel: [_ _ w436] -> w411
                tunnel: [_ _ w435] -> w410
                tunnel: [_ _ w434] -> w409
                tunnel: [_ _ w433] -> w408
                tunnel: [_ _ w432] -> w407
                tunnel: [_ _ w431] -> w406
                tunnel: [_ _ w430] -> w405
                tunnel: [_ _ w429] -> w404
                tunnel: [_ _ w428] -> w403
                tunnel: [_ _ w427] -> w402
                tunnel: [_ _ w426] -> w401
                tunnel: [_ _ w425] -> w400
                tunnel: [_ _ w424] -> w399
                tunnel: [_ _ w423] -> w398
                tunnel: [_ _ w422] -> w397
                tunnel: [_ _ w420] -> w396
                frame 0 {
                  n180 = One Button Dialog(message="해당하는 나사가 없음.\n관리자에게 문의바람." ("메시지")) -> ()  [unwired: 1 in, 1 out]
                }
                frame Default {
                  n181 = One Button Dialog(message="두개 이상의 나사가 검색됨.\n관리자에게 문의바람." ("메시지")) -> ()  [unwired: 1 in, 1 out]
                }
                frame 1 {
                  n182 = Index Array(array=w438) -> (element #1=w420:string, element #2=w424:string, element #3=w423:string, element #4=w425:string, element #5=w437:string, element #6=w436:string, element #7=w435:string, element #8=w434:string, element #9=w433:string, element #10=w432:string, element #11=w422:string, element #12=w431:string, element #13=w430:string, element #14=w421:string, element #15=w429:string, element #16=w428:string, element #17=w427:string, element #18=w426:string)  [unwired: 18 in]
                }
              }
            }
            frame True {
              w451 = "-"
              n183 = Index Array(array=w455) -> (element #1=w460:string, element #2=w459:string, element #3=w458:string)  [unwired: 3 in]
              n184 = case shown="\"M\"" w460 {
                tunnel: ["유니파이 나사" ("새 원소/부분배열") "관용 평행 나사" ("새 원소/부분배열") "미터 나사" ("새 원소/부분배열")] -> w441
                tunnel: w459 -> [w480 w504 w515]
                tunnel: [w474 w498 w515] -> w440
                tunnel: w458 -> [w478 w502 w514]
                tunnel: [w476 w500 w514] -> w453
                tunnel: ["60" "55" "60"] -> w452
                tunnel: [w468 w492 w511] -> w457
                tunnel: w450 -> [w467 _ _]
                tunnel: w449 -> [_ w491 _]
                tunnel: 0 ("비활성화된 인덱스 (열)") -> [w465 w489 _]
                tunnel: 1 ("비활성화된 인덱스 (열)") -> [w464 w488 _]
                frame Default {
                  w470 = 25.4 ("x")
                  n185 = Index Array(array=w467, index (col) #1=w464, index (col) #2=w465) -> (element #1=w463:string[], element #2=w466:string[])  [unwired: 2 in]
                  n186 = Search 1D Array(1D array=w466, element=w480) -> (index of element=w479:i32)  [unwired: 1 in]
                  n187 = Index Array(array=w463, index=w479) -> (element=w474:string)
                  n188 = case shown="기본" w478 {
                    selector: w478 -> [_ w484]
                    tunnel: [4.5 w483] -> w461
                    frame "4 1/2" {
                    }
                    frame Default {
                      n189 = Fract/Exp String To Number(string=w484) -> (number=w483:dbl)  [unwired: 3 in, 1 out]
                    }
                  }
                  n190 = Fract/Exp String To Number(string=w474) -> (number=w473:dbl)  [unwired: 3 in, 1 out]
                  n191 = Divide(x=0.649519, y=w461) -> (x/y=w471:dbl)
                  n192 = Divide(x=w470, y=w461) -> (x/y=w477:dbl)
                  n193 = Multiply(x=w470, y=w471) -> (x*y=w469:dbl)
                  n194 = Number To Fractional String(number=w477, precision (6)=i16 4 ("정밀도(6)")) -> (F-format string=w476:string)  [unwired: 2 in]
                  n195 = Subtract(x=w473, y=w469) -> (x-y=w468:dbl)
                }
                frame "G", "PF" {
                  w494 = 25.4 ("x")
                  n196 = Index Array(array=w491, index (col) #1=w488, index (col) #2=w489) -> (element #1=w487:string[], element #2=w490:string[])  [unwired: 2 in]
                  n197 = Search 1D Array(1D array=w490, element=w504) -> (index of element=w503:i32)  [unwired: 1 in]
                  n198 = Index Array(array=w487, index=w503) -> (element=w498:string)
                  n199 = case shown="기본" w502 {
                    selector: w502 -> [_ w508]
                    tunnel: [4.5 w507] -> w485
                    frame "4 1/2" {
                    }
                    frame Default {
                      n200 = Fract/Exp String To Number(string=w508) -> (number=w507:dbl)  [unwired: 3 in, 1 out]
                    }
                  }
                  n201 = Fract/Exp String To Number(string=w498) -> (number=w497:dbl)  [unwired: 3 in, 1 out]
                  n202 = Divide(x=0.640327 ("y"), y=w485) -> (x/y=w495:dbl)
                  n203 = Divide(x=w494, y=w485) -> (x/y=w501:dbl)
                  n204 = Multiply(x=w494, y=w495) -> (x*y=w493:dbl)
                  n205 = Number To Fractional String(number=w501, precision (6)=i16 4 ("정밀도(6)")) -> (F-format string=w500:string)  [unwired: 2 in]
                  n206 = Subtract(x=w497, y=w493) -> (x-y=w492:dbl)
                }
                frame "M" {
                  n207 = Fract/Exp String To Number(string=w515) -> (number=w510:dbl)  [unwired: 3 in, 1 out]
                  n208 = Fract/Exp String To Number(string=w514) -> (number=w513:dbl)  [unwired: 3 in, 1 out]
                  n209 = Multiply(x=w513, y=0.649519) -> (x*y=w509:dbl)
                  n210 = Subtract(x=w510, y=w509) -> (x-y=w511:dbl)
                }
              }
              n211 = Index Array(array=w455) -> (element #1=w446:string, element #2=w445:string, element #3=w444:string, element #4=w443:string, element #5=w442:string)  [unwired: 5 in]
              n212 = Number To Fractional String(number=w457, precision (6)=i16 4 ("정밀도(6)")) -> (F-format string=w454:string)  [unwired: 2 in]
            }
          }
          n213 = Build Array(w371, w373, w372, w374, w389, w388, w387, w386, w385, w384, w382, w381, w380, w379, w378, w377, w376, w375) -> (w383:string[])
        }
        n214 = Index Array(array=w361) -> (element #1=→"검색결과 1":string[], element #2=→"검색결과 2":string[])  [unwired: 4 in]
        n215 = call "Enq Msg.vi"("에러 입력(에러 없음)"=w366, "메세지"="측정력적용", "큐 입력"=w364) -> ("에러 출력"=w365:errorcluster)  [unwired: 7 in, 1 out]
      }
      frame "측정력적용" {
        w526 = "%#f" ("포맷 문자열")
        n216 = local read "검색결과 1"() -> (w538:string[])
        n217 = Index Array(array=w538, index #2=10 ("인덱스")) -> (element #1=w540:string, element #2=w539:string)  [unwired: 1 in]
        n218 = case shown="\"M\"" w540 {
          tunnel: [0 2] -> w537
          frame Default {
          }
          frame "M" {
          }
        }
        n219 = Fract/Exp String To Number(string=w539) -> (number=w536:dbl)  [unwired: 3 in, 1 out]
        n220 = property on="측정력" class="CmbBox"(error in=w549) -> (error out=w547:errorcluster, "Strings And Values[]"=w548:T5)  [unwired: 1 in, 1 out]
        n221 = Delete From Array(array=dbl[][] [[0.2, 0.5, 0.318, 0.529, 1.67, 2.26, 4.0, 6.0], [0.6, 1.0, 0.577, 1.058, 4.41, 5.39, 4.0, 6.0], [1.25, 4.0, 1.27, 4.233, 8.83, 10.79, 6.0, 8.0], [4.5, 6.0, 5.08, 6.35, 8.83, 10.79, 8.0, 10.0]], length=2, index (col)=w537) -> (array with subset deleted=w535:dbl[][])  [unwired: 1 in, 1 out]
        n222 = for {
          tunnel: w536 -> [w561]
          tunnel: w535 -> [w562] mode=indexing
          tunnel: [w557] -> w529
          tunnel: [w550] -> w528
          tunnel: [w552] -> w527
          tunnel: [w551] -> w525
          stop <- w560 stop-if-true
          n223 = Index Array(array=w562) -> (element #1=w558:dbl, element #2=w559:dbl, element #3=w557:dbl, element #4=w550:dbl, element #5=w554:dbl, element #6=w553:dbl)  [unwired: 6 in]
          n224 = In Range and Coerce(upper limit=w559, x=w561, lower limit=w558) -> (In Range?=w560:bool)  [unwired: 1 out]
          n225 = Build Array(w550, w557) -> (w556:dbl[])
          n226 = Build Array(w554, w553) -> (w555:dbl[])
          n227 = call "Standard Deviation.vi"("X"=w556) -> ("mean"=w552:dbl)  [unwired: 8 in, 2 out]
          n228 = call "Standard Deviation.vi"("X"=w555) -> ("mean"=w551:dbl)  [unwired: 8 in, 2 out]
        }
        n229 = Format Into String(format string=w526, w527) -> (resulting string=w524:string)  [unwired: 2 in, 1 out]
        n230 = Format Into String(format string=w526, w525) -> (resulting string=w523:string)  [unwired: 2 in, 1 out]
        n231 = for {
          tunnel: w548 -> [w570] mode=indexing
          tunnel: w528 -> [w569]
          tunnel: w529 -> [w568]
          tunnel: [w565] -> w541
          stop <- w566 stop-if-true
          n232 = Unbundle By Name(w570) -> ("Value"=w565:string)
          n233 = Fract/Exp String To Number(string=w565) -> (number=w567:dbl)  [unwired: 3 in, 1 out]
          n234 = In Range and Coerce(upper limit=w569, x=w567, lower limit=w568) -> (In Range?=w566:bool)  [unwired: 1 out]
        }
        n235 = Build Array(w524, w523) -> (w522:string[])
        n236 = Format Into String(format string="(%.3f ~ %.3f) N" ("포맷 문자열"), w529, w528) -> (resulting string=→"Force":string)  [unwired: 2 in, 1 out]
        n237 = property on="측정력" class="CmbBox"(error in=w547, "Value"=w541) -> (error out=w545:errorcluster)  [unwired: 1 in, 1 out]
        n238 = To Variant(anything=w522) -> (Variant=w542:variant)
        n239 = call "Enq Msg.vi"("에러 입력(에러 없음)"=w545, "값"=w542, "메세지"="Condition적용", "큐 입력"=w543) -> ("에러 출력"=w544:errorcluster)  [unwired: 6 in, 1 out]
      }
      frame "Condition적용" {
        n240 = local read "검색결과 1"() -> (w590:string[])
        n241 = local read "검색결과 2"() -> (w605:string[])
        n242 = local read "형태"() -> (w601:enum16{"GO/NOT GO", "GO", "NOT GO"})
        n243 = Variant To Data(error in=w577, type=string[] [], Variant=w576) -> (data=w573:string[], error out=w574:errorcluster)
        n244 = Equal To 0?(x=w601) -> (x = 0?=w600:bool)
        n245 = Select(t=2, s=w600, f=1) -> (s? t:f=w597:i32)
        n246 = Index Array(array=w590, index #1=9 ("인덱스")) -> (element #1=w591:string, element #2=w588:string)  [unwired: 1 in]
        n247 = Build Array(w590, w605) -> (w607:string[][])
        n248 = Fract/Exp String To Number(string=w591) -> (number=w589:dbl)  [unwired: 3 in, 1 out]
        n249 = Fract/Exp String To Number(string=w588) -> (number=w587:dbl)  [unwired: 3 in, 1 out]
        n250 = local read "Condition 1"() -> (w610:string[][])
        n251 = local read "Condition 2"() -> (w606:string[][])
        n252 = xnode ("수식 2")("E0"=w589, "P"=w587) -> ("결과"=w593:dbl)  [unwired: 1 in, 1 out]
        n253 = Index Array(array=w573) -> (element #1=w572:string, element #2=w571:string)  [unwired: 2 in]
        n254 = Build Array(w610, w606) -> (w609:string[][][])
        n255 = local read "Resolution 1"() -> (w579:string[][])
        n256 = Quotient & Remainder(x=w593, y=1.0) -> (x-y*floor(x/y)=w595:dbl, floor(x/y)=w583:dbl)
        n257 = Multiply(x=w595, y=60.0 ("x")) -> (x*y=w582:dbl)
        n258 = Index Array(array=w579, index (col)=3 ("비활성화된 인덱스 (열)")) -> (element=w578:string[])  [unwired: 1 in]
        n259 = Format Into String(format string="%d˚ %d´" ("포맷 문자열"), w583, w582) -> (resulting string=w581:string)  [unwired: 2 in, 1 out]
        n260 = for {
          N: w597 -> [_]
          tunnel: w609 -> [w628] mode=indexing
          tunnel: w607 -> [w647] mode=indexing
          tunnel: [w630] -> w608 mode=indexing
          tunnel: w581 -> [w629]
          tunnel: w578 -> [w626]
          tunnel: w572 -> [w622]
          tunnel: w571 -> [w621]
          w623 = 7 ("비활성화된 인덱스 (열)")
          w638 = "0" ("f")
          n261 = Replace Array Subset(array=w628, new element #1=w629, index (row) #1=4 ("인덱스 (행)"), index (col) #1=w623, new element #2=w622, index (row) #2=10 ("인덱스 (행)"), index (col) #2=w623, new element #3=w621, index (row) #3=12 ("인덱스 (행)"), index (col) #3=w623) -> (w627:string[][])
          n262 = Index Array(array=w647, index #1=8 ("인덱스")) -> (element #1=w637:string, element #2=w636:string, element #3=w635:string, element #4=w644:string)  [unwired: 3 in]
          n263 = Equal?(x=w644, y="55") -> (x = y?=w642:bool)
          n264 = Select(t="27.5" ("y"), s=w642, f="30") -> (s? t:f=w639:string)
          n265 = Build Array(w637, w637, w636, w635, w635, w635, w635, w635, w635, w635, w639, w639, w639, w639) -> (w646:string[])
          n266 = Build Array(w637, w637, w636, w635, w635, w635, w635, w635, w635, w635, w638, w638, w638, w638) -> (w633:string[])
          n267 = for {
            tunnel: w627 -> [w654] mode=indexing
            tunnel: [w653] -> w630 mode=indexing
            tunnel: w646 -> [w651] mode=indexing
            tunnel: 3 ("비활성화된 인덱스 (열)") -> [w652]
            tunnel: w633 -> [w650] mode=indexing
            tunnel: 5 ("비활성화된 인덱스 (열)") -> [w649]
            tunnel: w626 -> [w648] mode=indexing
            n268 = Replace Array Subset(array=w654, new element #1=w651, index #1=w652, new element #2=w650, index #2=w649, new element #3=w648) -> (w653:string[])  [unwired: 1 in]
          }
        }
        n269 = Index Array(array=w608) -> (element #1=→"Condition 1":string[][], element #2=→"Condition 2":string[][])  [unwired: 6 in]
        n270 = call "Enq Msg.vi"("에러 입력(에러 없음)"=w574, "메세지"="SPEC적용", "큐 입력"=w602) -> ("에러 출력"=w603:errorcluster)  [unwired: 7 in, 1 out]
      }
      frame "SPEC적용" {
        n271 = local read "Resolution 1"() -> (w677:string[][])
        n272 = local read "Condition 1"() -> (w655:string[][])
        n273 = local read "검색결과 1"() -> (w687:string[])
        n274 = local read "검색결과 2"() -> (w686:string[])
        n275 = local read "형태"() -> (w673:enum16{"GO/NOT GO", "GO", "NOT GO"})
        n276 = global read "Global_Cal Info.vi" "Func List"() -> (w679:string[][])
        n277 = Equal To 0?(x=w673) -> (x = 0?=w672:bool)
        n278 = call "Variables Data IO.vi"("Select"=Cmd_Var_Data_IO."Spec Default", "error in"=w683, "Func_ext"=w682) -> ("error out"=w666:errorcluster, "Data Out"=w681:string[][], "Func_ext Out"=w662:string)  [unwired: 6 in]
        n279 = Select(t=2, s=w672, f=1) -> (s? t:f=w669:i32)
        n280 = Build Array(w687, w686) -> (w688:string[][])
        n281 = Empty Array?(array=w681) -> (empty?=w680:bool)
        n282 = case shown="거짓" w680 {
          tunnel: w688 -> [w694 w747]
          tunnel: [w693 w748] -> w685
          tunnel: w681 -> [_ w749]
          tunnel: w679 -> [_ w746]
          tunnel: string[] ["바깥지름", "바깥지름", "유효지름", "피치", "피치", "피치", "피치", "피치", "피치", "피치", "반각", "반각", "반각", "반각"] ("추가된 배열") -> [_ w745]
          tunnel: w677 -> [w692 w744]
          tunnel: w669 -> [w691 w743]
          tunnel: [w690 w742] -> w657
          tunnel: [w689 w741] -> w656
          tunnel: w655 -> [_ w740]
          frame True {
            n283 = for {
              N: w691 -> [_]
              tunnel: w694 -> [w712] mode=indexing
              tunnel: [w700] -> w693 mode=indexing
              tunnel: w692 -> [w698]
              tunnel: [w696] -> w690 mode=indexing
              tunnel: [w695] -> w689 mode=indexing
              w703 = "-" ("문자열")
              n284 = Index Array(array=w712, index #1=5 ("인덱스"), index #3=12 ("인덱스")) -> (element #1=w696:string, element #2=w695:string, element #3=w711:string, element #4=w709:string, element #5=w710:string, element #6=w708:string, element #7=w706:string, element #8=w705:string)  [unwired: 6 in]
              n285 = Concatenate Strings(w703, w706) -> (w704:string)
              n286 = Concatenate Strings(w703, w705) -> (w702:string)
              n287 = Build Array(w709, w709, w708, w704, w704, w704, w704, w704, w704, w704, w702, w702, w702, w702) -> (w701:string[])
              n288 = Build Array(w711, w711, w710, w706, w706, w706, w706, w706, w706, w706, w705, w705, w705, w705) -> (w707:string[])
              n289 = for {
                tunnel: string[] ["μm", "μm", "μm", "μm", "μm", "μm", "μm", "μm", "μm", "μm", "´", "´", "´", "´"] ("추가된 배열") -> [w720] mode=indexing
                tunnel: w698 -> [w725] mode=indexing
                tunnel: w707 -> [w722] mode=indexing
                tunnel: w701 -> [w721] mode=indexing
                tunnel: [w714] -> w700 mode=indexing
                n290 = Index Array(array=w725, index #1=2 ("인덱스")) -> (element #1=w723:string, element #2=w719:string)  [unwired: 1 in]
                n291 = call "Number Format.vi"("입력값"=w723) -> ("정밀도(단위적용)"=w718:i32)  [unwired: 10 in]
                n292 = case shown="기본" w721 {
                  selector: w721 -> [_ w728]
                  tunnel: w720 -> [_ w731]
                  tunnel: w719 -> [_ w730]
                  tunnel: ["-" ("환산값 (string)") w729] -> w717
                  tunnel: w718 -> [_ w727]
                  frame "-", "--" {
                  }
                  frame Default {
                    n293 = call "Unit Conversion.vi"("소수점 자리수"=w727, "환산단위"=w730, "입력단위"=w731, "입력값"=w728) -> ("환산값 (string)"=w729:string)  [unwired: 2 in, 5 out]
                  }
                }
                n294 = case shown="기본" w722 {
                  selector: w722 -> [_ w736]
                  tunnel: w720 -> [_ w739]
                  tunnel: w719 -> [w732 w738]
                  tunnel: ["-" ("환산값 (string)") w737] -> w716
                  tunnel: w718 -> [_ w735]
                  tunnel: [w732 w734] -> w715
                  frame "-", "--" {
                  }
                  frame Default {
                    n295 = call "Unit Conversion.vi"("소수점 자리수"=w735, "환산단위"=w738, "입력단위"=w739, "입력값"=w736) -> ("환산단위"=w734:string, "환산값 (string)"=w737:string)  [unwired: 2 in, 4 out]
                  }
                }
                n296 = Build Array(w717, w716, w715) -> (w714:string[])
              }
            }
          }
          frame False {
            n297 = for {
              N: w743 -> [_]
              tunnel: w747 -> [w777] mode=indexing
              tunnel: w749 -> [w779]
              tunnel: [w758] -> w748 mode=indexing
              tunnel: w746 -> [w761]
              tunnel: w745 -> [w760]
              tunnel: w744 -> [w759]
              tunnel: [w755] -> w742 mode=indexing
              tunnel: [w754] -> w741 mode=indexing
              tunnel: w740 -> [w753]
              w752 = 10 ("인덱스")
              n298 = Index Array(array=w761) -> (element=w765:string[])  [unwired: 2 in]
              n299 = Index Array(array=w777, index #1=5 ("인덱스"), index #4=w752) -> (element #1=w755:string, element #2=w754:string, element #3=w776:string, element #4=w775:string)  [unwired: 2 in]
              n300 = Index Array(array=w753, index (row) #1=w752, index (col) #1=3 ("비활성화된 인덱스 (열)"), index (col) #2=4 ("비활성화된 인덱스 (열)")) -> (element #1=w750:string, element #2=w770:string[])  [unwired: 1 in]
              n301 = Build Array(w776, w776, w776, w775, w775, w775, w775, w775, w775, w775, w750, w750, w750, w750) -> (w757:string[])
              n302 = Index Array(array=w765) -> (element #1=w774:string, element #3=w773:string)  [unwired: 3 in, 1 out]
              n303 = Index Array(array=w759, index (col)=3 ("비활성화된 인덱스 (열)")) -> (element=w768:string[])  [unwired: 1 in]
              n304 = for {
                tunnel: w774 -> [w801]
                tunnel: [w800] -> w767 mode=indexing
                tunnel: w773 -> [w799]
                tunnel: "" ("원소") -> [w798]
                tunnel: w760 -> [w797] mode=indexing
                tunnel: w757 -> [w794] mode=indexing
                tunnel: w770 -> [w793] mode=indexing
                tunnel: w768 -> [w792] mode=indexing
                tunnel: [w791] -> w762 mode=indexing
                n305 = call "Unit Conversion.vi"("환산단위"=w792, "입력단위"=w793, "입력값"=w794) -> ("환산단위"=w795:string, "환산값 (DBL)"=w791:dbl, "환산값 (string)"=w796:string)  [unwired: 3 in, 3 out]
                n306 = Build Array(w801, w799, w797, w798, w798, w796, w795) -> (w800:string[])
              }
              n307 = call "Match_Spec.vi"("DATA IN"=w767, "SPEC IN"=w779) -> ("Spec Out"=w778:string[][])  [unwired: 7 in, 2 out]
              n308 = call "Spec Calculation.vi"("기준값 열번호"=5 ("열번호(기준값)"), "Resolution"=w759, "Condition in"=w767, "Spec Default"=w778) -> ("Spec (DBL)"=w764:dbl[][], "Spec out"=w763:string[][])  [unwired: 6 in]
              n309 = for {
                tunnel: w764 -> [w787] mode=indexing
                tunnel: w763 -> [w784] mode=indexing
                tunnel: w762 -> [w786] mode=indexing
                tunnel: [w780] -> w758 mode=indexing
                n310 = Subtract(x=w787, y=w786) -> (x-y=w785:dbl[])
                n311 = for {
                  tunnel: w785 -> [w790] mode=indexing
                  tunnel: [w788] -> w782 mode=indexing
                  n312 = Format Into String(format string="%#f" ("포맷 문자열"), w790) -> (resulting string=w788:string)  [unwired: 2 in, 1 out]
                }
                n313 = Index Array(array=w784, index=2 ("인덱스")) -> (element=w781:string)
                n314 = Build Array (concatenate)(w782, w781) -> (w780:string[])
              }
            }
          }
        }
        n315 = Index Array(array=w657) -> (element #1=→"구분 1":string, element #2=→"구분 2":string)  [unwired: 2 in]
        n316 = Index Array(array=w656) -> (element #1=→"종류 1":string, element #2=→"종류 2":string)  [unwired: 2 in]
        n317 = Index Array(array=w685) -> (element #1=w665:string[][], element #2=w664:string[][])  [unwired: 6 in]
        "Spec 1" <- w665
        "Spec 2" <- w664
        n318 = Build Array (concatenate)(w665, w664) -> (w663:string[][])
        n319 = call "Variables Data IO.vi"("Select"=Cmd_Var_Data_IO."Spec", "error in"=w666, "Data In"=w663, "Func_ext"=w662) -> ("error out"=w667:errorcluster)  [unwired: 5 in, 2 out]
        n320 = call "Enq Msg.vi"("에러 입력(에러 없음)"=w667, "메세지"="CALSTD적용", "큐 입력"=w674) -> ("에러 출력"=w675:errorcluster)  [unwired: 7 in, 1 out]
      }
      frame "CALSTD적용" {
        (unwired) enum32{"큰 값", "가까운 값"}."가까운 값" ("dw조건")
        w818 = 0 ("인덱스 (행)")
        n321 = local read "검색결과 1"() -> (w834:string[])
        n322 = Index Array(array=w834, index #1=7 ("인덱스"), index #2=10 ("인덱스"), index #4=0 ("인덱스")) -> (element #1=w832:string, element #2=w807:string, element #3=w813:string)  [unwired: 1 in, 1 out]
        n323 = for {
          tunnel: w835 -> [w851]
          tunnel: [w852] -> w829 mode=indexing
          tunnel: string[] ["바깥지름", "바깥지름", "유효지름", "피치", "피치", "피치", "피치", "피치", "피치", "피치", "반각", "반각", "반각", "반각"] ("추가된 배열") -> [w850] mode=indexing
          tunnel: w832 -> [w848]
          tunnel: w807 -> [w847]
          tunnel: w813 -> [w842]
          i -> [w849]
          n324 = Equal?(x=w842, y="55") -> (x = y?=w846:bool)
          n325 = Select(t="27.5" ("y"), s=w846, f="30") -> (s? t:f=w841:string)
          n326 = case shown="10.." w849 {
            tunnel: [w858 w864 w870] -> w852
            tunnel: w851 -> [w857 w863 w869]
            tunnel: w850 -> [w856 w862 w868]
            tunnel: w848 -> [w854 _ _]
            tunnel: w847 -> [_ w859 _]
            tunnel: w841 -> [_ _ w865]
            frame 0..2 {
              w855 = ""
              n327 = Build Array(w857, w857, w856, w855, w855, w854, "mm" ("원소")) -> (w858:string[])
            }
            frame Default {
              w861 = ""
              n328 = Build Array(w863, w863, w862, w861, w861, w859, "mm" ("원소")) -> (w864:string[])
            }
            frame 10.. {
              w867 = ""
              n329 = Build Array(w869, w869, w868, w867, w867, w865, "˚" ("원소")) -> (w870:string[])
            }
          }
        }
        n330 = call "Variables Data IO.vi"("Select"=Cmd_Var_Data_IO."CMC Default", "error in"=w840, "Func_ext"=w835) -> ("error out"=w839:errorcluster, "Data Out"=w836:string[][], "Func_ext Out"=w838:string)  [unwired: 6 in]
        n331 = Build Array (concatenate)(w829, w829) -> (w814:string[][])
        n332 = call "Match_CMC.vi"("CMC IN"=w836, "error in"=w839, "Condition IN"=w814, "Func_ext"=w838) -> ("error out"=w826:errorcluster, "Func_ext out"=w827:string)  [unwired: 4 in, 2 out]
        n333 = Delete From Array(array=w814, length=2 ("길이"), index (col)=5 ("비활성화된 인덱스 (열)")) -> (deleted portion=w821:string[][])  [unwired: 1 in, 1 out]
        n334 = Format Into String("dw조건") -> (resulting string=w803:string)  [unwired: 3 in, 1 out]
        n335 = call "Variables Data IO.vi"("Select"=Cmd_Var_Data_IO."Condition Default", "error in"=w826, "Data In"=w821, "Func_ext"=w827) -> ("error out"=w825:errorcluster, "Func_ext Out"=w824:string)  [unwired: 5 in, 1 out]
        n336 = call "STD Cal Data.vi"("error in"=w825, "문자열"=w803, "Func_ext"=w824) -> ("error out"=w808:errorcluster, "Data Out"=w820:string[][])  [unwired: 4 in, 3 out]
        n337 = Index Array(array=w820, index (row) #1=w818, index (col) #1=13 ("인덱스 (행)"), index (row) #2=w818, index (col) #2=16 ("인덱스 (행)")) -> (element #1=w806:string, element #2=w816:string)
        n338 = Format Into String(format string="%s %s" ("포맷 문자열"), w806, w816) -> (resulting string=→"3 wire":string)  [unwired: 2 in, 1 out]
        n339 = To Variant(anything=w806) -> (Variant=w805:variant)
        n340 = call "Enq Msg.vi"("에러 입력(에러 없음)"=w808, "값"=w805, "메세지"="조건변경", "큐 입력"=w810) -> ("에러 출력"=w811:errorcluster)  [unwired: 6 in, 1 out]
      }
      frame "조건변경" {
        w880 = 0 ("비활성화된 인덱스 (페이지)")
        w879 = 3 ("인덱스 (행)")
        n341 = local read "형태"() -> (w902:enum16{"GO/NOT GO", "GO", "NOT GO"})
        n342 = Variant To Data(error in=w898, type="", Variant=w897) -> (data=w887:string, error out=w875:errorcluster)
        n343 = Equal To 0?(x=w902) -> (x = 0?=w901:bool)
        n344 = Select(t=2, s=w901, f=1) -> (s? t:f=w905:i32)
        n345 = local read "Condition 1"() -> (w904:string[][])
        n346 = local read "Condition 2"() -> (w903:string[][])
        n347 = property on="형태" class="Enum (엄격한)"(error in=w875) -> (error out=w874:errorcluster, "Strings []"=w873:string[], "Value"=w872:enum16{"GO/NOT GO", "GO", "NOT GO"})  [unwired: 1 in, 1 out]
        n348 = Build Array(w904, w903) -> (w906:string[][][])
        n349 = Index Array(array=w873, index=w872) -> (element=w871:string)
        n350 = Index Array(array=w906, index (dim 0) #1=w880, index (dim 1) #1=10 ("인덱스 (행)"), index (dim 2) #1=w879, index (dim 0) #2=w880, index (dim 1) #2=w879, index (dim 2) #2=w879, index (dim 0) #3=w880, index (dim 1) #3=2 ("인덱스 (행)"), index (dim 2) #3=w879) -> (element #1=w885:string, element #2=w882:string, element #3=w877:string)
        n351 = local read "측정력"() -> (w888:string)
        n352 = Fract/Exp String To Number(string=w885) -> (number=w884:dbl)  [unwired: 3 in, 1 out]
        n353 = Fract/Exp String To Number(string=w882) -> (number=w881:dbl)  [unwired: 3 in, 1 out]
        n354 = Fract/Exp String To Number(string=w877) -> (number=w876:dbl)  [unwired: 3 in, 1 out]
        n355 = Fract/Exp String To Number(string=w887) -> (number=w886:dbl)  [unwired: 3 in, 1 out]
        n356 = for {
          N: w905 -> [_]
          tunnel: w906 -> [w918] mode=indexing
          tunnel: [w921] -> w896 mode=indexing
          tunnel: [w921] -> w890 mode=concatenating
          tunnel: w888 -> [w920]
          tunnel: w886 -> [w919]
          tunnel: w884 -> [w917]
          tunnel: w881 -> [w916]
          tunnel: w876 -> [w915]
          tunnel: w871 -> [w908]
          w910 = 2 ("인덱스 (행)")
          n357 = xnode "수식"("a½"=w917, "P"=w916, "E0"=w915, "dw"=w919, "dm"=w919) -> ("결과"=w913:dbl)  [unwired: 1 in, 1 out]
          n358 = Number To Fractional String(number=w913, precision (6)=i16 4 ("정밀도(6)")) -> (F-format string=w911:string)  [unwired: 2 in]
          n359 = Replace Array Subset(array=w918, new element #1=w920, index (row) #1=7 ("인덱스 (행)"), index (col) #1=7 ("비활성화된 인덱스 (열)"), new element #2=w911, index (row) #2=w910, index (col) #2=5 ("비활성화된 인덱스 (열)"), new element #3=w908, index (row) #3=w910, index (col) #3=0 ("비활성화된 인덱스 (열)")) -> (w921:string[][])
        }
        n360 = Index Array(array=w896) -> (element #1=w895:string[][], element #2=w894:string[][])  [unwired: 6 in]
        n361 = local write "Condition 1"(w895) -> ()
        n362 = local write "Condition 2"(w894) -> ()
        n363 = call "Variables Data IO.vi"("Select"=Cmd_Var_Data_IO."Condition", "error in"=w874, "Data In"=w890, "Func_ext"=w891) -> ("error out"=w892:errorcluster)  [unwired: 5 in, 2 out]
      }
    }
  }
  n364 = control-ref of="dw조건"() -> ()  [unwired: 1 out]
  n365 = Release Queue(queue=w10, error in (no error)=w11) -> (error out=w8:errorcluster)  [unwired: 1 in, 2 out]
  n366 = Merge Errors(w9, w8) -> (→"에러 출력":errorcluster)
